vi "Write Selection Start[].vi"(8 "error in (no error)":errorcluster, 10 "SelStart[]":u32[](array[numeric]), 11 "Array.lvclass in":refnum<class "Array.lvclass">) -> (0 "error out":errorcluster, 3 "Array.lvclass out":refnum<class "Array.lvclass">)   [LabVIEW 2015, in "Array.lvclass"]
uses:
  Array.lvclass
  Array.lvclass/Array.ctl
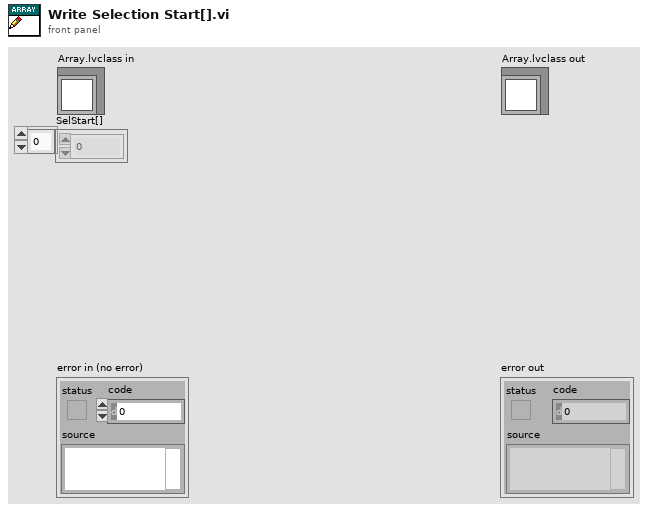
[diagram p1: front panel]
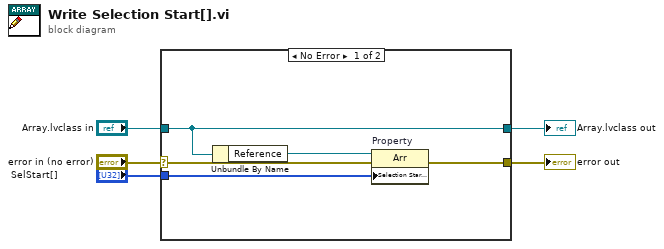
[diagram p0: block diagram]
diagram:
  n1 = case shown="No Error" "error in (no error)" {
    selector: "error in (no error)" -> [w6 w12]
    tunnel: [w10 w12] -> w4
    tunnel: [w8 w11] -> w2
    tunnel: "Array.lvclass in" -> [w8 w11]
    tunnel: "SelStart[]" -> [w9 _]
    frame No Error {
      n2 = Unbundle By Name(w8) -> ("Reference"=w7:refnum<vi>)
      n3 = property on="Property" class="Arr"(reference=w7, error in=w6, "Selection Start []"=w9) -> (error out=w10:errorcluster)  [unwired: 1 out]
    }
    frame Error {
    }
  }
  "error out" <- w4
  "Array.lvclass out" <- w2
